vi "题目6.vi"   [LabVIEW 2017]
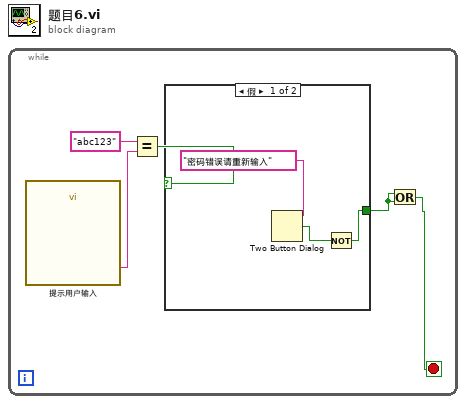
[diagram p0: block diagram]
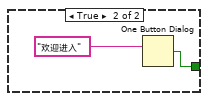
[diagram p2: hidden frame]
diagram:
  n1 = while {
    stop <- w2 stop-if-true
    n2 = call "提示用户输入"() -> ("请输入密码"=w3:string)  [unwired: 16 in, 3 out]
    n3 = Equal?(x="abc123", y=w3) -> (x = y?=w4:bool)
    n4 = case shown="假" w4 {
      tunnel: [w6 w9] -> w1
      frame False {
        n5 = Two Button Dialog(message="密码错误请重新输入") -> (T button?=w7:bool)  [unwired: 2 in]
        n6 = Not(x=w7) -> (.not. x?=w6:bool)
      }
      frame True {
        n7 = One Button Dialog(message="欢迎进入") -> (true=w9:bool)  [unwired: 1 in]
      }
    }
    n8 = Or(x=w1, y=w1) -> (x .or. y?=w2:bool)
  }
